vi "RedefineMasterIP.vi"() -> (0 "Abort?":bool)   [LabVIEW 2012]
uses:
  <userlib>/ROSforLV/ROS/Code/_ROSDefinition.vi
panel:
  in  "Cancel Button":bool
  in  "OK Button":bool
  in  "Port":string
  in  "Address":string
  # "Please enter your Master IP address."
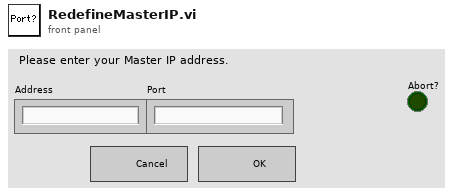
[diagram p1: front panel]
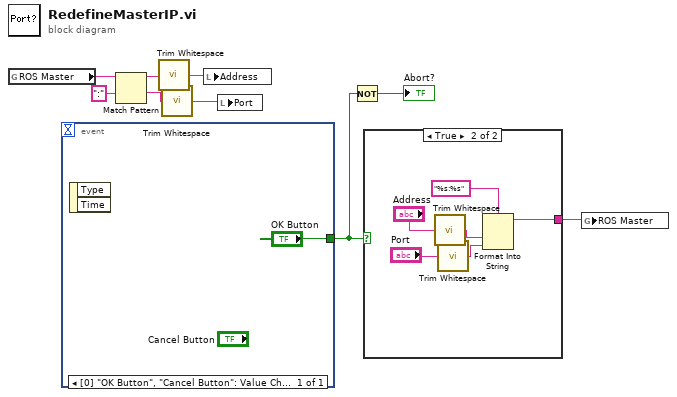
[diagram p0: block diagram]
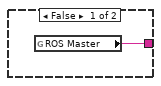
[diagram p2: hidden frame]
diagram:
  n1 = global read "_ROSDefinition.vi" "ROS Master"() -> (w9:string)
  n2 = event shown="[0] \"OK Button\", \"Cancel Button\": Value Change;  Panel Close" {
    selector: _ -> [_]
    dyn-events: _ -> [_]
    timeout: _ -> [_]
    tunnel: ["OK Button"] -> w3
    event "OK Button", "Cancel Button": Value Change; Panel Close {
      n3 = event-data() -> ()  [unwired: 1 in, 2 out]
    }
  }
  n4 = Match Pattern(string=w9, regular expression=":") -> (before substring=w7:string, after substring=w4:string)  [unwired: 1 in, 2 out]
  n5 = call <vilib>:"Trim Whitespace.vi"("string"=w7) -> ("trimmed string"=w6:string)  [unwired: 1 in]
  n6 = call <vilib>:"Trim Whitespace.vi"("string"=w4) -> ("trimmed string"=w5:string)  [unwired: 1 in]
  n7 = local write "Address"(w6) -> ()
  n8 = local write "Port"(w5) -> ()
  n9 = Not(x=w3) -> (.not. x?=→"Abort?":bool)
  n10 = case shown="True" w3 {
    tunnel: [w11 w12] -> w2
    frame False {
      n11 = global read "_ROSDefinition.vi" "ROS Master"() -> (w11:string)
    }
    frame True {
      n12 = call <vilib>:"Trim Whitespace.vi"("string"="Address") -> ("trimmed string"=w14:string)  [unwired: 1 in]
      n13 = call <vilib>:"Trim Whitespace.vi"("string"="Port") -> ("trimmed string"=w13:string)  [unwired: 1 in]
      n14 = Format Into String(format string="%s:%s", w14, w13) -> (resulting string=w12:string)  [unwired: 2 in, 1 out]
    }
  }
  n15 = global write "_ROSDefinition.vi" "ROS Master"(w2) -> ()
